vi "qREC STATE.vi"(0 "System no.":i32=1 min=1 max=4 step=1, 2 "RecorderIDs to query":string[](array[string]), 5 "error in":errorcluster) -> (14 "Data Recorder State":T1[](array[typedef]), 19 "error out":errorcluster)   [LabVIEW 2020]
doc: "REC? STATE (Get Data Recorder State)\n\nDescription\nQueries the state of the data recorders of the controller.\nThe state of a data recorder determines whether the data recorder is configurable or can record \ndata.\n\nFormat\nREC? STATE[ <RecorderID>]\n\nArguments\nREC? STATE without arguments queries all data recorders of the controller.\n<RecorderID>\nData recorder, whose state is to be queried; to be specified as alias (p. 94) \nThe available data recorders can be queried with USG? SYS (p. 80). \nPossible values: REC_1 to RECn, where n = number of data recorders in the controller\n\nResponse\n{<RecorderID> = <RecorderStatus> LF}\n<RecorderStatus>\nCurrent state of the data recorder\nDescriptions of the states can be queried with USG? PROP (p. 79). For further details, see the \nstate diagram for the data recorder (p. 110). \nPossible values: RUN, CFG, WAIT\n\nExample \n>>REC? STATE\n<<REC_1=CFG\n<<REC_2=CFG\n>>REC? STATE REC_2\n<<REC_2=CFG\n\nNotes\nFor further details, see \"Data Recorder - GCS 3.0\" (p. 107). \n\nUser command level\nUSR"
uses:
  RecorderStatus.ctl
panel:
  # "REC? STATE (Get Data Recorder State)\n\nQueries the state of the data recorders of the controller.\nThe state of a data recorder determines whether the data recorder is configurable or can record data."
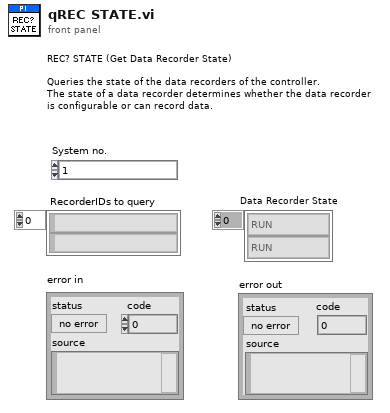
[diagram p1: front panel]
types:
  T1 = typedef "RecorderStatus.ctl" = enum16{"RUN", "CFG", "WAIT"}
  T2 = typedef "Syntax.ctl" = enum16{"GCS 1.0", "GCS 2.0", "GCS 3.0"}
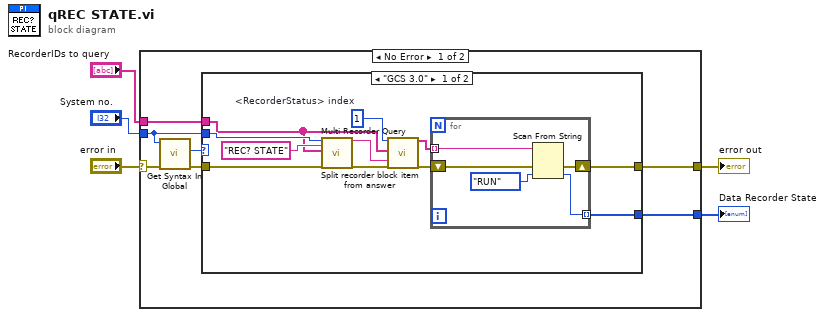
[diagram p0: block diagram]
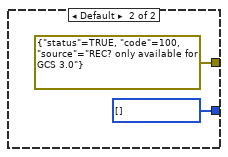
[diagram p2: hidden frame]
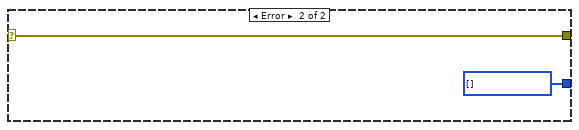
[diagram p3: hidden frame]
diagram:
  n1 = case shown="No Error" "error in" {
    selector: "error in" -> [w12 w32]
    tunnel: [w9 w32] -> w4
    tunnel: "RecorderIDs to query" -> [w7 _]
    tunnel: "System no." -> [w6 _]
    tunnel: [w8 w31] -> w3
    frame No Error {
      n2 = call "Get Syntax In Global.vi"("error in"=w12, "System no."=w6) -> ("error out"=w10:errorcluster, "Syntax"=w11:T2)  [unwired: 8 in]
      n3 = case shown="\"GCS 3.0\"" w11 {
        tunnel: w10 -> [w21 _]
        tunnel: [w14 errorcluster {"status"=TRUE, "code"=100, "source"="REC? only available for GCS 3.0"} ("error out")] -> w9
        tunnel: [w13 w29] -> w8
        tunnel: w7 -> [w19 _]
        tunnel: w6 -> [w23 _]
        frame "GCS 3.0" {
          w20 = 1  # <RecorderStatus> index
          n4 = call "Multi Recorder Query.vi"("System no."=w23, "Recorder Command"="REC? STATE" ("format string"), "RecorderIDs to query"=w19, "error in"=w21) -> ("Answer"=w18:string, "error out"=w17:errorcluster)  [unwired: 14 in]
          n5 = call "Split recorder block item from answer.vi"("Slice block item"=w20, "RecorderIDs to query"=w19, "Input string"=w18, "error in"=w17) -> ("Sliced text segments"=w16:string[], "error out"=w15:errorcluster)  [unwired: 14 in]
          n6 = for {
            tunnel: w16 -> [w25] mode=indexing
            shift-right: [w26] -> w14
            shift-left: w15 -> [w27]
            tunnel: [w24] -> w13 mode=indexing
            n7 = Scan From String(input string=w25, error in=w27, default 1=RecorderStatus."RUN" ("RecorderStatus")) -> (error out=w26:errorcluster, output 1=w24:T1)  [unwired: 2 in, 2 out]
          }
        }
        frame Default {
          w29 = T1[] [] items=["RUN", "CFG", "WAIT"] ("Data Recorder State")
        }
      }
    }
    frame Error {
      w31 = T1[] [] items=["RUN", "CFG", "WAIT"] ("Data Recorder State")
    }
  }
  "error out" <- w4
  "Data Recorder State" <- w3
